vi "Obtain Msg Q.vi"(10 "Alias":string) -> (0 "error out":errorcluster, 3 "Msg Queue out":refnum<class "Msg Q.lvclass">)   [LabVIEW 2021, in "LVCAM.lvlib" / "Msg Q.lvclass"]
uses:
  Msg Q.lvclass
  Msg/Msg.lvclass
  Msg Q.lvclass/Msg Q.ctl
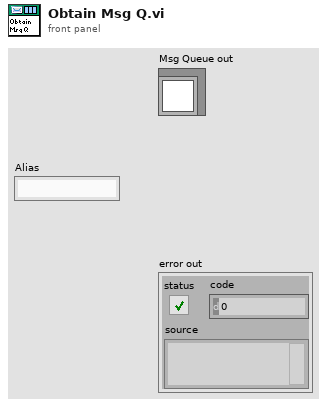
[diagram p1: front panel]
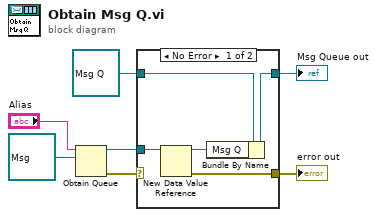
[diagram p0: block diagram]
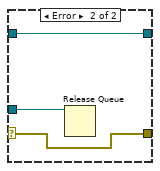
[diagram p2: hidden frame]
diagram:
  n1 = Obtain Queue(name (unnamed)="Alias", element data type=refnum<class "Msg.lvclass"> refnum ("Artifex Actor Model.lvlib:Msg.lvclass")) -> (queue out=w4:refnum<queue>, error out=w5:errorcluster)  [unwired: 3 in, 1 out]
  n2 = case shown="No Error" w5 {
    selector: w5 -> [_ w13]
    tunnel: refnum<class "Msg Q.lvclass"> refnum ("Msg Queue out") -> [w12 w15]
    tunnel: w4 -> [w11 w14]
    tunnel: [w9 w15] -> w3
    tunnel: [w8 w13] -> w1
    frame No Error {
      n3 = New Data Value Reference(data value=w11) -> (data value reference=w10:refnum<data-value>, error out=w8:errorcluster)  [unwired: 1 in]
      n4 = Bundle By Name(cluster=w12, "Msg Q"=w10) -> (w9:refnum<class "Msg Q.lvclass">)
    }
    frame Error {
      n5 = Release Queue(queue=w14) -> ()  [unwired: 2 in, 3 out]
    }
  }
  "Msg Queue out" <- w3
  "error out" <- w1
